vi "Add (Elementwise) - R,RM.vi"(1 "Real Matrix A":T1, 2 "Real Scalar c":dbl) -> (0 "c + A":T1)   [LabVIEW 2020, in "NI_Matrix.lvlib"]
doc: "Computes the sum of the inputs."
uses:
  <vilib>/Analysis/Matrix/NI_Matrix.lvlib
  <vilib>/Analysis/Matrix/Datatypes/RealMatrix.ctl
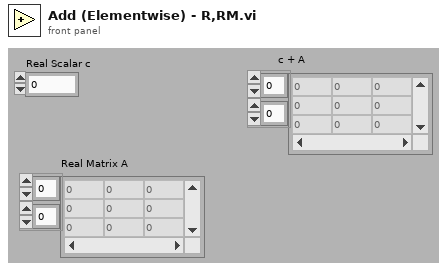
[diagram p1: front panel]
types:
  T1 = typedef "NI_Matrix.lvlib/RealMatrix.ctl" = dbl[][]
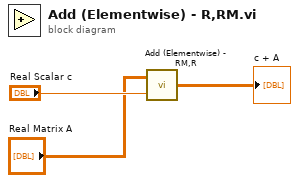
[diagram p0: block diagram]
diagram:
  n1 = call <vilib>:"Add (Elementwise) - RM,R.vi"("Real Scalar c"="Real Scalar c", "Real Matrix A"="Real Matrix A") -> ("A + c"=→"c + A":T1)
